vi "Experimental VI.vi"() -> ()   [LabVIEW 2016]
panel:
  out "unsigned 16bit integer":u16
  out "Power % Gauge":dbl(knob) scale=0.0..100.0
  in  "Power %":dbl min=0.0 max=100.0 step=0.5 format="%.1f"
  in  "stop":bool
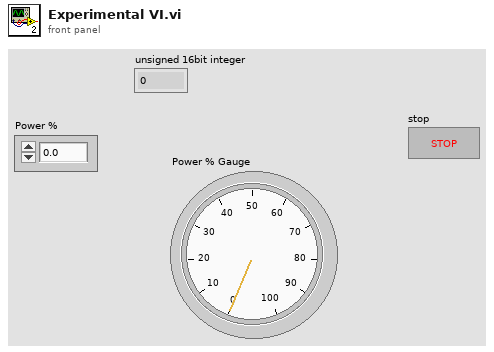
[diagram p1: front panel]
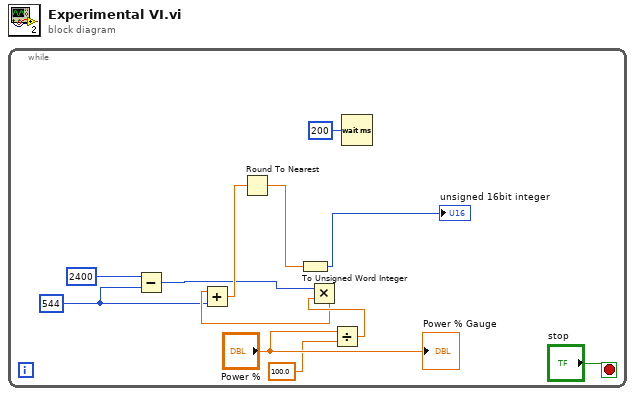
[diagram p0: block diagram]
diagram:
  n1 = while {
    stop <- "stop" stop-if-true
    w1 = 544
    n2 = Subtract(x=2400, y=w1) -> (x-y=w3:i32)
    n3 = Divide(x="Power %", y=100.0) -> (x/y=w6:dbl)
    n4 = Multiply(x=w3, y=w6) -> (x*y=w5:dbl)
    n5 = Add(x=w5, y=w1) -> (x+y=w4:dbl)
    n6 = Round To Nearest(number=w4) -> (nearest integer value=w9:dbl)
    n7 = To Unsigned Word Integer(number=w9) -> (unsigned 16bit integer=→"unsigned 16bit integer":u16)
    n8 = Wait (ms)(milliseconds to wait=u32 200) -> ()  [unwired: 1 out]
    "Power % Gauge" <- "Power %"
  }
